vi "Create Parameters Array.vi"(8 "error in (no error)":errorcluster, 9 "Initial Settings":variant, 11 "Initial Parameters":cluster{T1[]}[](array[cluster])) -> (0 "error out":errorcluster, 3 "Initial Parameters":cluster{T1[]}[](array[cluster]))   [LabVIEW 2015, in "Diagnostics Addon Engine.lvlib" / "Inline Async API.lvlib"]
uses:
  Inline Async API.lvlib
  Controls/Parameters Cluster.ctl
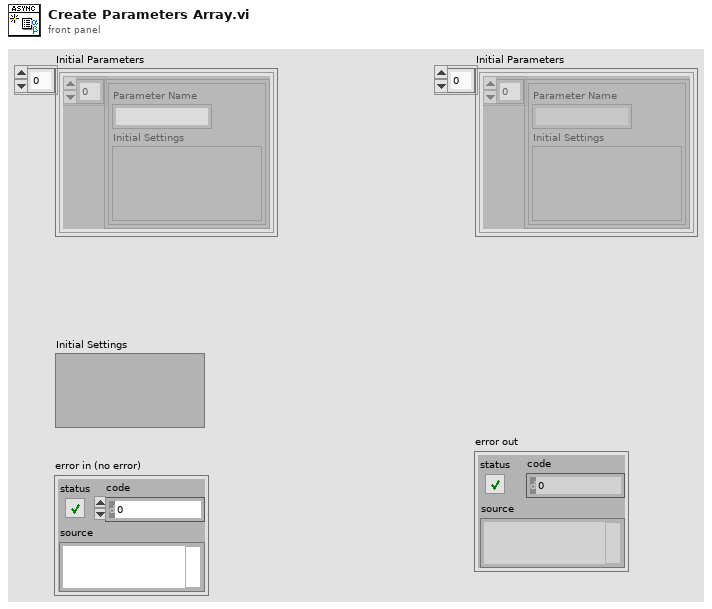
[diagram p1: front panel]
types:
  T1 = typedef "Diagnostics Addon Engine.lvlib/Inline Async API.lvlib/Parameters Cluster.ctl" = cluster{"Parameter Name":string, "Initial Settings":variant}
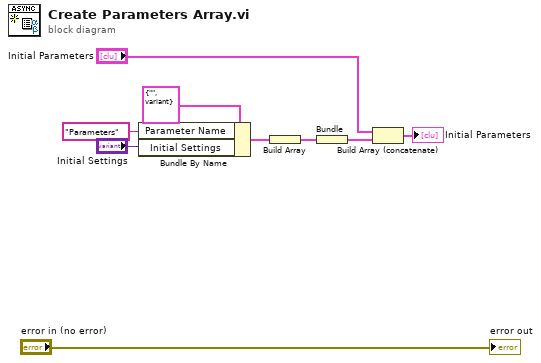
[diagram p0: block diagram]
diagram:
  n1 = Bundle By Name(cluster=T1 {"Parameter Name"="", "Initial Settings"=variant} ("Parameters"), "Parameter Name"="Parameters", "Initial Settings"="Initial Settings") -> (w5:T1)
  n2 = Build Array(w5) -> (w9:T1[])
  n3 = Bundle ("Display and Log Process Parameters")(w9) -> (w8:cluster{T1[]})  [unwired: 1 in]
  n4 = Build Array (concatenate)("Initial Parameters", w8) -> (→"Initial Parameters":cluster{T1[]}[])
  "error out" <- "error in (no error)"
